vi "Station Close.vi"(8 "error in (no error)":errorcluster, 11 "Station in":refnum<class "Station.lvclass">) -> (0 "error out":errorcluster, 3 "Station out":refnum<class "Station.lvclass">)   [LabVIEW 2018, in "Station.lvclass"]
uses:
  Station.lvclass
  Station Support/Controls/Server Control.ctl
  Station.lvclass/Station.ctl
panel:
  out "Currently Closing Instrument:":string
  # "Model Number:\nInstrument Number:\nRack ID:\nInst Mnemonic:\nComp Mnemonic:\nSubsys Mnemonic:\nIP Address:\nSub Address:\nFirmware Rev:\nExpected Options:\nRequired Options: \nExcluded Options:"
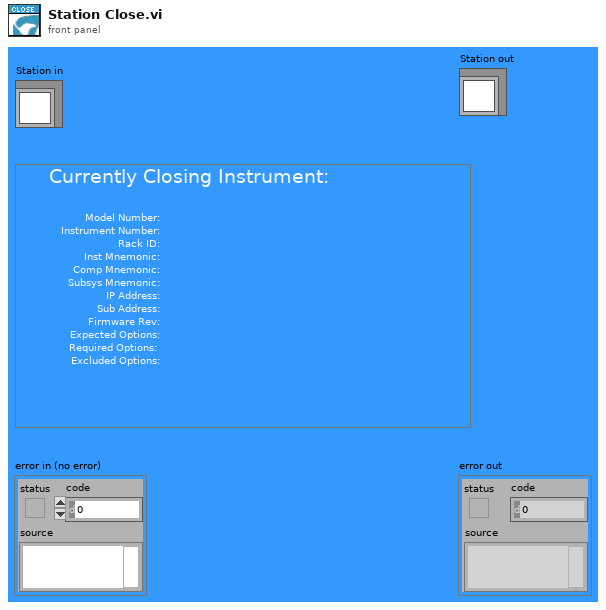
[diagram p1: front panel]
types:
  T1 = typedef "Server Control.ctl" = enum16{"Open New Reference", "Remove Reference", "Kill Server", "Set Station Ref", "Get Station Ref"}
  T2 = enum16{"Open New Reference", "Remove Reference", "Kill Server"}
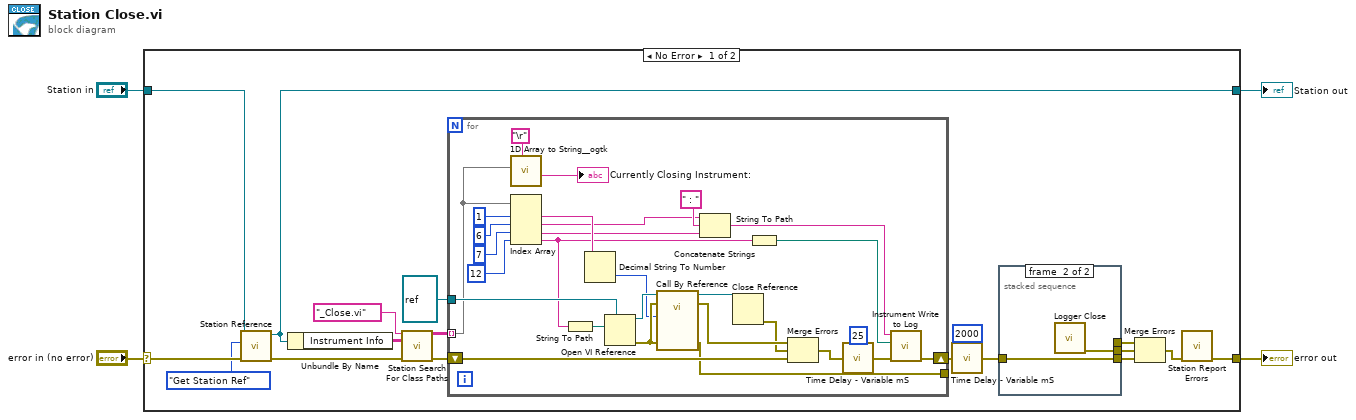
[diagram p0: block diagram]
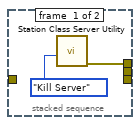
[diagram p2: hidden frame]
diagram:
  n1 = case shown="No Error" "error in (no error)" {
    selector: "error in (no error)" -> [w10 w56]
    tunnel: [w17 w56] -> w3
    tunnel: "Station in" -> [w7 w55]
    tunnel: [w8 w55] -> w2
    frame No Error {
      n2 = call "Station Reference.vi"("error in (no error)"=w10, "Action (0: Create)"=Server_Control."Get Station Ref", "Station in"=w7) -> ("error out"=w9:errorcluster, "Station out"=w8:refnum<class "Station.lvclass">)  [unwired: 7 in]
      n3 = Unbundle By Name(w8) -> ("Instrument Info"=w12:string[][])
      n4 = call "Station Search For Class Paths.vi"("VI select"="_Close.vi", "Instrument Info"=w12, "error in (no error)"=w9) -> ("Updated Inst Info"=w21:string[][], "error out"=w22:errorcluster)  [unwired: 11 in]
      n5 = for {
        tunnel: w21 -> [w44] mode=indexing
        shift-right: [w34] -> w20
        shift-left: w22 -> [w46]
        tunnel: refnum<vi> refnum ("VI Refnum") -> [w54]
        tunnel: [w45] -> _
        n6 = call <userlib>:"1D Array to String__ogtk.vi"("delimiter (Tab)"="\r", "Array of Strings"=w44) -> ("delimited string"=→"Currently Closing Instrument:":string)  [unwired: 9 in]
        n7 = Index Array(array=w44, index #1=1 ("index"), index #2=6 ("index"), index #3=7 ("index"), index #4=12 ("index")) -> (element #1=w42:string, element #2=w32:string, element #3=w31:string, element #4=w30:string)
        n8 = String To Path(string=w30) -> (path=w51:path)
        n9 = Decimal String To Number(string=w42) -> (number=w41:i32)  [unwired: 2 in, 1 out]
        n10 = Open VI Reference(type specifier VI Refnum (for type only)=w54, vi path=w51) -> (vi reference=w52:refnum<vi>, error out=w53:errorcluster)  [unwired: 4 in]
        n11 = call-by-ref "?"(reference=w52, error in=w53, "User Reference"=w41, "error in (no error)"=w53) -> (reference out=w48:refnum<vi>, error out=w49:errorcluster, 19:"error out"=w45:errorcluster)  [unwired: 17 in]
        n12 = Concatenate Strings(w32, " : " ("string"), w31) -> (w29:string)
        n13 = Close Reference(reference=w48) -> (error out=w47:errorcluster)  [unwired: 1 in]
        n14 = String To Path(string=w30) -> (path=w28:path)
        n15 = Merge Errors(w49, w47, w46) -> (w50:errorcluster)
        n16 = call "Time Delay - Variable mS.vi"("milliseconds to wait"=u32 25, "error in (no error)"=w50) -> ("error out"=w35:errorcluster)  [unwired: 2 in]
        n17 = call "Instrument Write to Log.vi"("error in (no error)"=w35, "Current VI's Path"=w28, "Insstrument Address"=w29) -> ("error out"=w34:errorcluster)  [unwired: 8 in]
      }
      n18 = call "Time Delay - Variable mS.vi"("milliseconds to wait"=u32 2000, "error in (no error)"=w20) -> ("error out"=w19:errorcluster)  [unwired: 2 in]
      n19 = stacked-sequence {
        tunnel: w19 -> [_ w26]
        tunnel: [w23 _] -> w14
        tunnel: [_ w26] -> w15
        tunnel: [_ w25] -> w13
        frame #0 {
          n20 = call "Station Class Server Utility.vi"("Action (0: Create)"=T2."Kill Server") -> ("error out"=w23:errorcluster)  [unwired: 10 in]
        }
        frame #1 {
          n21 = call "Logger Close.vi"() -> ("error out"=w25:errorcluster)  [unwired: 15 in]
        }
      }
      n22 = Merge Errors(w14, w13, w15) -> (w16:errorcluster)
      n23 = call "Station Report Errors.vi"("error in (no error)"=w16) -> ("error out"=w17:errorcluster)  [unwired: 10 in]
    }
    frame Error {
    }
  }
  "error out" <- w3
  "Station out" <- w2
